vi "Get 3D Live Position Offset.vi"(3 "Mode":T5, 5 "Traverse line In":T2 {"Carrier_2 Q (l/min)" format="%#.2f"; "Row Duration (mins)" format="%#.1f"; "Row No" min=0; "Trace Gas Concentration (%)" min=0.0 format="%#_4f"; "Carrier_1 Q (l/min)" format="%#.2f"; "Tunnel Speed" format="%#.2f"; "Start X" format="%#.2f"; "Start Y" format="%#.2f"; "Start Z" format="%#.2f"; "End X" format="%#.2f"; "End Y" format="%#.2f"; "End Z" format="%#.2f"; "Averaging time (min)" min=0.0 format="%#.2f"}) -> (0 "Error Message":string, 1 "Status":T1, 2 "Traverse line Out":T2 {"Carrier_2 Q (l/min)" format="%#.2f"; "Row Duration (mins)" format="%#.1f"; "Row No" min=0; "Trace Gas Concentration (%)" min=0.0 format="%#_4f"; "Carrier_1 Q (l/min)" format="%#.2f"; "Tunnel Speed" format="%#.2f"; "Start X" format="%#.2f"; "Start Y" format="%#.2f"; "Start Z" format="%#.2f"; "End X" format="%#.2f"; "End Y" format="%#.2f"; "End Z" format="%#.2f"; "Averaging time (min)" min=0.0 format="%#.2f"})   [LabVIEW 2017]
uses:
  Gen Trav/Traverse_cluster.ctl
  Gen Trav/Spacing.ctl
  Controls/Multi_run_mode.ctl
  Controls/User_Specific_mode.ctl
  Gen Trav/Multi_Run_Status.ctl
  Controls/Setup.ctl
  Controls/Save_Data.ctl
  Camera Server/Camera enum/Camera resolution.ctl
  Globals/Trav_pos_global.vi
  Globals/Meas_global.vi
panel:
  out "Vertical Offset":sgl
  # "X           Y            Z"
  # "Start"
  # "End"
  # "X           Y            Z"
  # "Start"
  # "End"
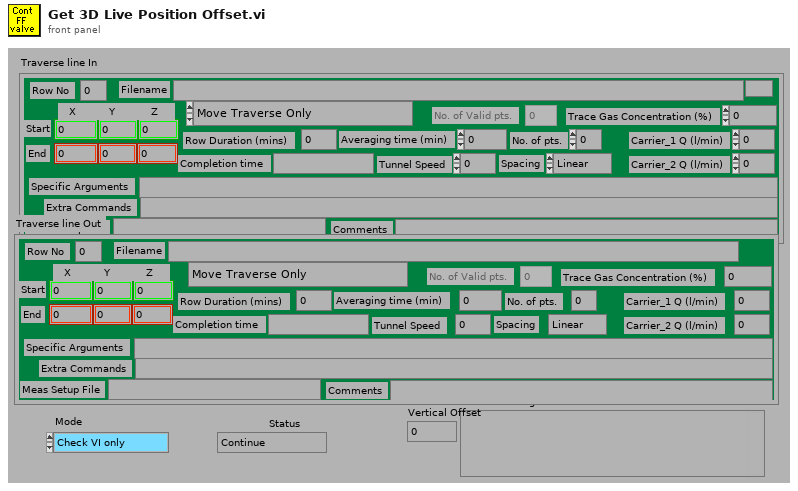
[diagram p1: front panel]
types:
  T1 = typedef "Multi_Run_Status.ctl" = enum16{"Continue", "Continue with Error", "Jump to Next Point", "Jump to Next Row", "Jump To Fall Back", "Terminate Run"}
  T2 = typedef "Traverse_cluster.ctl" = cluster{"Start X":sgl, "Start Y":sgl, "Start Z":sgl, "End X":sgl, "End Y":sgl, "End Z":sgl, "No. of pts.":i32, "Spacing":T3, "Filename":path, "Tunnel Speed":dbl, "Averaging time (min)":dbl, "Extra Commands":string, "Carrier_1 Q (l/min)":dbl, "Carrier_2 Q (l/min)":dbl, "Trace Gas Concentration (%)":dbl, "Specific Arguments":string, "Comments":string, "Row No":i32, "Row Type Selector":T4, "Completion time":string, "Row Duration (mins)":dbl, "No. of Valid pts.":i32, "Meas Setup File":string}
  T3 = typedef "Spacing.ctl" = enum16{"Linear", "Log", "Gauss", "Specified", "N/A"}
  T4 = typedef "Multi_run_mode.ctl" = enum16{"Move Traverse Only", "Set Tunnel Speed Only", "Set Source Only", "Set Measurement Conditions", "Single Measurement", "Vertical Profile", "Lateral Profile", "Longitudinal Profile", "Explore Volume", "Multi-Axis Profile", "Auto Calibrate", "Meas Fast FID Bkgnd", "Check Beam Power", "Scanning Valve Measurement", "Run VI Named:", "Set ADAM Ch", "Wait (minutes)", "Send Message", "Synchronize With:", "Fall Back to this Row", "Turn Off Row Repeating", "Blank Row", "Traverse 3D Volume"}
  T5 = typedef "User_Specific_mode.ctl" = enum16{"Check VI only", "Run VI"}
  T6 = enum16{"To Traverse Coordinates", "To User Coordinates"}
  T7 = typedef "Save_Data.ctl" = enum16{"Save No Data", "Save Data"}
  T8 = typedef "Setup.ctl" = enum16{"Run Program", "Show Setup", "Save Current Setup", "Setup Front Panel"}
  T9 = typedef "Tunnel_Coordinates.ctl" = enum16{"Work in Tunnel Coordinates", "Work in Model Coordinates"}
  T10 = typedef "Status_Cluster.ctl" = cluster{"Status":T1, "Error Type":string, "Error Description":string}
  T11 = typedef "Camera resolution.ctl" = u8
  T12 = typedef "Analysis_info_cluster.ctl" = cluster{"Colour":u32, "Inst type":T13, "Inst name":string, "Symbol":string, "Code name":string, "Extra Info":string, "Inst Array":T14, "Extra Titles":string[], "Extra Values":string[], "U":dbl, "u^2":dbl, "u^3":dbl, "u^4":dbl, "Skew_u":dbl, "Kurt_u":dbl, "Sd Error in Mean":dbl, "% u'/U":dbl, "X":dbl, "Y":dbl, "Z":dbl, "Timescale integral Estimate":dbl, "Sd Error in Variance":dbl, "Calib File":path, "Calib Constants":dbl[], "Output Position":bool, "Full Stats":bool, "Av Sampling Rate":dbl, "Av No of Samples":dbl, "Total Meas Time (s)":dbl, "ADAM Ch Name":string, "Max value":dbl, "Min value":dbl}
  T13 = typedef "Inst_type.ctl" = enum16{"Propeller anemometer", "Raw voltage", "Pressure Transducer", "Pitot-static tube", "Preston tube", "Hot wire", "Cross wire 1", "Cross wire 2", "Generic Linear", "Generic Polynomial", "Generic BackPoly", "Fast FID", "Thermocouple", "Cold wire", "Pulsed Wire", "LDA Vel", "LDA Tran time", "LDA Arr time", "Microphone"}
  T14 = typedef "Instrument_Array.ctl" = enum16{"PWA", "LDA", "Analogue"}
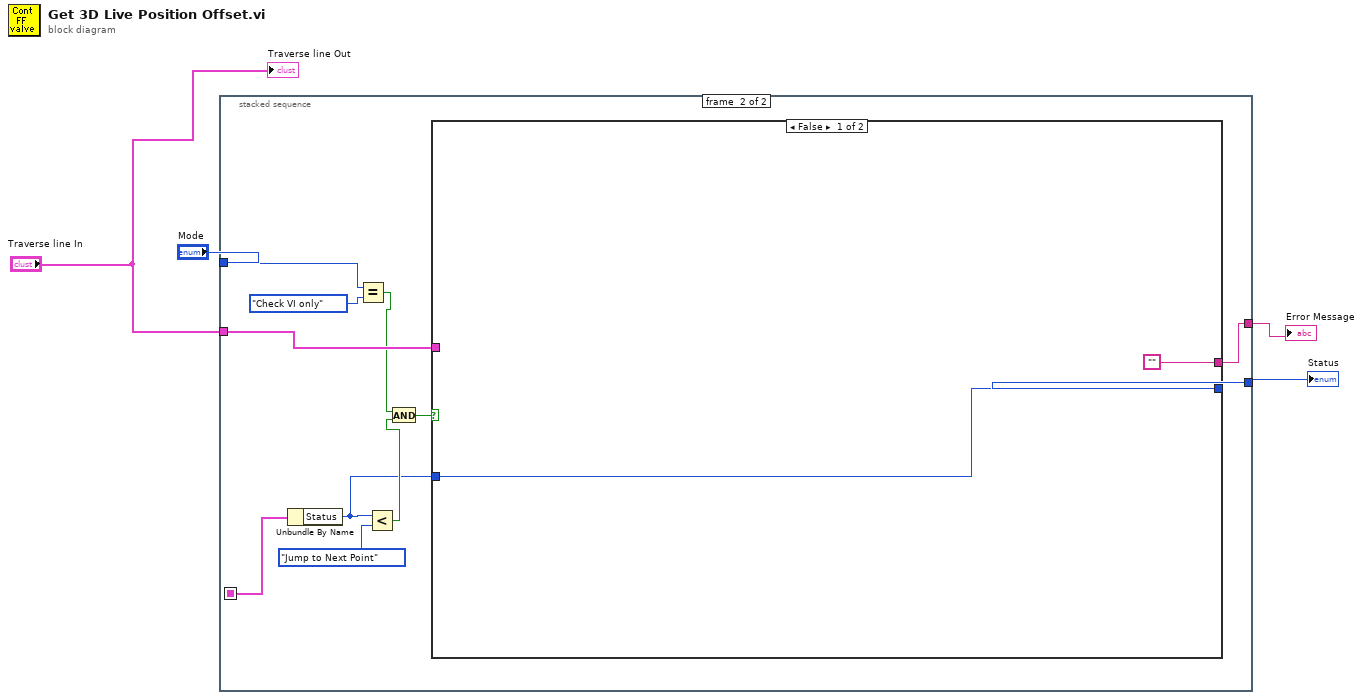
[diagram p0: block diagram]
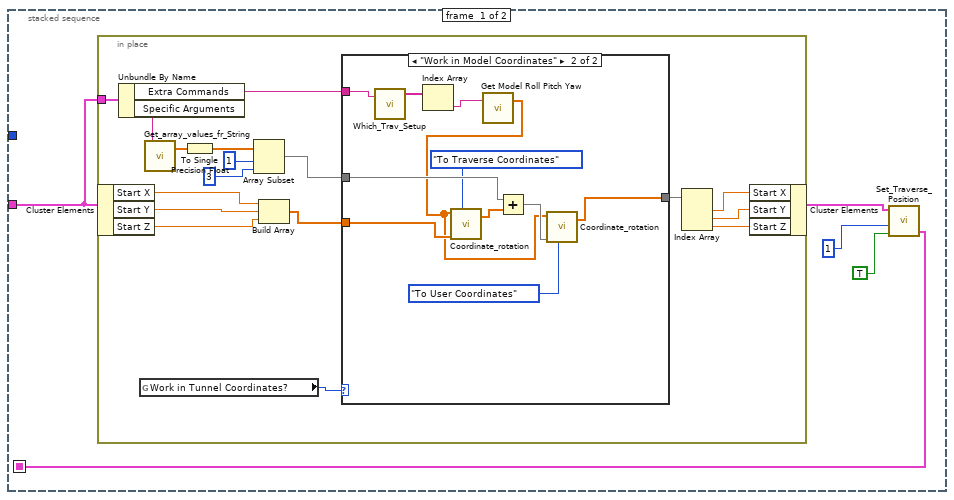
[diagram p2: hidden frame]
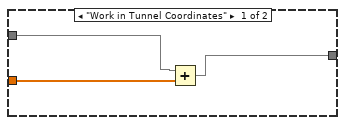
[diagram p3: hidden frame]
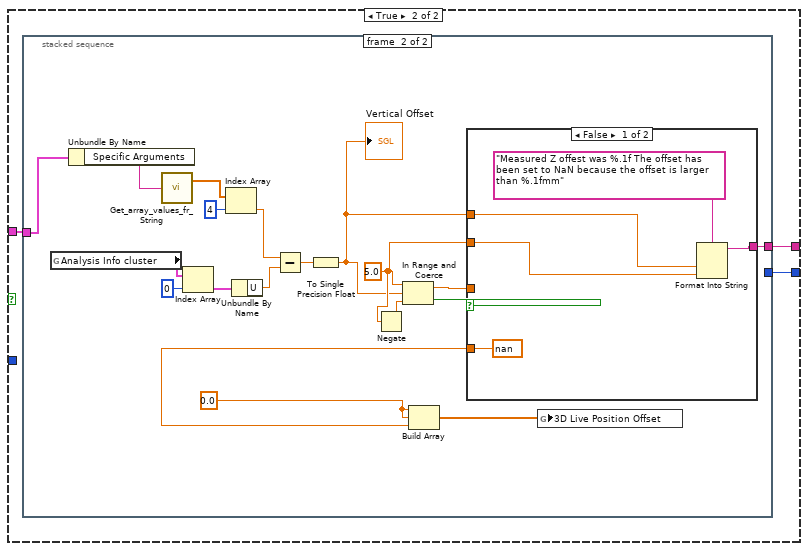
[diagram p4: hidden frame]
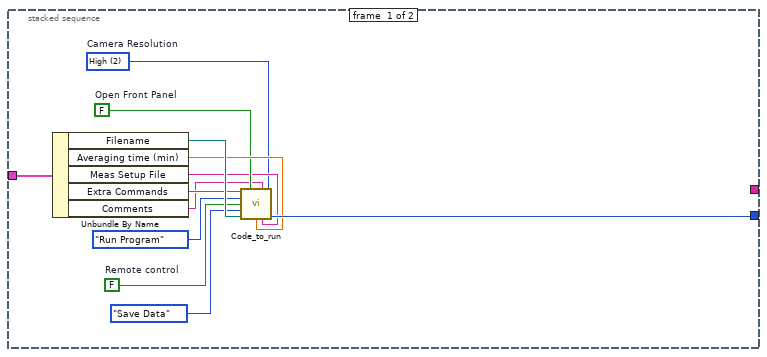
[diagram p5: hidden frame]
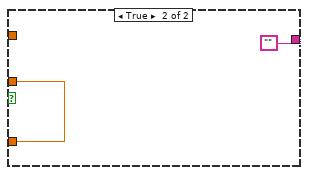
[diagram p6: hidden frame]
diagram:
  n1 = stacked-sequence {
    seq-local: [w6 _] -> [_ w50]
    tunnel: [_ w41] -> w4
    tunnel: "Traverse line In" -> [w5 w51]
    tunnel: "Mode" -> [_ w47]
    tunnel: [_ w43] -> w1
    frame #0 {
      n2 = in-place {
        in-place-border: w5 -> [w12]
        n3 = in-place-cluster #1(w5) -> ("Start X"=w24:sgl, "Start Y"=w23:sgl, "Start Z"=w22:sgl)
        n4 = Unbundle By Name(w12) -> ("Extra Commands"=w10:string, "Specific Arguments"=w11:string)
        n5 = global read "Trav_pos_global.vi" "Work in Tunnel Coordinates?"() -> (w26:T9)
        n6 = call "Get_array_values_fr_String.vi"("String Value"=w11) -> ("Numeric Array"=w25:dbl[])  [unwired: 1 out]
        n7 = To Single Precision Float(number=w25) -> (single precision float=w14:sgl[])
        n8 = Array Subset(array=w14, index=1, length=3) -> (w20:sgl[])
        n9 = Build Array(w24, w23, w22) -> (w19:sgl[])
        n10 = case shown="\"Work in Model Coordinates\"" w26 {
          tunnel: w20 -> [w29 w38]
          tunnel: w19 -> [w28 w40]
          tunnel: [w27 w36] -> w18
          tunnel: w10 -> [_ w31]
          frame "Work in Tunnel Coordinates" {
            n11 = Add(x=w29, y=w28) -> (x+y=w27:sgl[])
          }
          frame "Work in Model Coordinates" {
            n12 = call "Which_Trav_Setup.vi"("Extra Command String"=w31) -> ("Traverse Setups"=w33:string[])  [unwired: 1 in, 2 out]
            n13 = Index Array(array=w33) -> (element=w32:string)  [unwired: 1 in]
            n14 = call "Get Model Roll Pitch Yaw.vi"("Traverse Name"=w32) -> ("Model:    Roll        Pitch         Yaw  (deg)"=w30:sgl[])  [unwired: 1 in, 1 out]
            n15 = call "Coordinate_rotation.vi"("Roll-Pitch-Yaw"=w30, "Input Position"=w40, "Mode"=T6."To Traverse Coordinates") -> ("Output Position"=w39:sgl[])  [unwired: 2 in, 1 out]
            n16 = Add(x=w38, y=w39) -> (x+y=w37:sgl[])
            n17 = call "Coordinate_rotation.vi"("Roll-Pitch-Yaw"=w30, "Input Position"=w37, "Mode"=T6."To User Coordinates") -> ("Output Position"=w36:sgl[])  [unwired: 2 in, 1 out]
          }
        }
        n18 = Index Array(array=w18) -> (element #1=w17:sgl, element #2=w16:sgl, element #3=w15:sgl)  [unwired: 3 in]
        n19 = in-place-cluster #1("Start X"=w17, "Start Y"=w16, "Start Z"=w15) -> (w7:T2)
      }
      n20 = call "Set_Traverse_Position.vi"("Last Part of Move?"=TRUE, "Currently on Point"=1, "Traverse line"=w7) -> ("Status Cluster"=w6:T10)  [unwired: 3 in]
    }
    frame #1 {
      n21 = Unbundle By Name(w50) -> ("Status"=w42:T1)
      n22 = Equal?(x=w47, y=User_Specific_mode."Check VI only" ("Mode")) -> (x = y?=w45:bool)
      n23 = Less?(x=w42, y=Multi_Run_Status."Jump to Next Point") -> (x < y?=w46:bool)
      n24 = And(x=w45, y=w46) -> (x .and. y?=w44:bool)
      n25 = case shown="False" w44 {
        tunnel: [w53 w56] -> w43
        tunnel: w51 -> [_ w55]
        tunnel: w42 -> [w53 _]
        tunnel: ["" w54] -> w41
        frame False {
        }
        frame True {
          n26 = stacked-sequence {
            tunnel: [w68 _] -> w56
            tunnel: w55 -> [w57 w71]
            tunnel: [_ w69] -> w54
            frame #0 {
              w58 = T11 2 items=["Low", "Med.", "High", "Max."]  # Camera Resolution
              w64 = FALSE  # Open Front Panel
              w66 = FALSE  # Remote control
              n27 = Unbundle By Name(w57) -> ("Filename"=w67:path, "Averaging time (min)"=w65:dbl, "Meas Setup File"=w61:string, "Extra Commands"=w60:string, "Comments"=w59:string)
              n28 = call "Code_to_run.vi"("Extra command String"=w60, "Open Front Panel"=w64, "Current Row Comments"=w59, "Camera Resolution"=w58, "setup"=Setup."Run Program", "Remote control"=w66, "File"=Save_Data."Save Data", "Results Filename"=w67, "Averaging time (min)"=w65, "Setup filename"=w61) -> ("Status"=w68:T1)  [unwired: 2 in, 3 out]
            }
            frame #1 {
              w72 = sgl 5.0 ("upper limit")
              w78 = sgl 0.0
              n29 = global read "Meas_global.vi" "Analysis Info cluster"() -> (w87:T12[])
              n30 = Unbundle By Name(w71) -> ("Specific Arguments"=w84:string)
              n31 = call "Get_array_values_fr_String.vi"("String Value"=w84) -> ("Numeric Array"=w82:dbl[])  [unwired: 1 out]
              n32 = Index Array(array=w87, index=0) -> (element=w85:T12)
              n33 = Index Array(array=w82, index=4) -> (element=w81:dbl)
              n34 = Unbundle By Name(w85) -> ("U"=w80:dbl)
              n35 = Subtract(x=w81, y=w80) -> (x-y=w77:dbl)
              n36 = To Single Precision Float(number=w77) -> (single precision float=w70:sgl)
              "Vertical Offset" <- w70
              n37 = Negate(x=w72) -> (-x=w76:sgl)
              n38 = In Range and Coerce(upper limit=w72, x=w70, lower limit=w76) -> (coerced(x)=w74:sgl, In Range?=w75:bool)
              n39 = case shown="False" w75 {
                tunnel: w70 -> [w92 _]
                tunnel: w74 -> [_ w93]
                tunnel: [w90 ""] -> w69
                tunnel: [sgl nan ("upper limit") w93] -> w73
                tunnel: w72 -> [w88 _]
                frame False {
                  n40 = Format Into String(format string="Measured Z offest was %.1f The offset has  been set to NaN because the offset is larger than %.1fmm", w92, w88) -> (resulting string=w90:string)  [unwired: 2 in, 1 out]
                }
                frame True {
                }
              }
              n41 = Build Array(w78, w78, w73) -> (w79:sgl[])
              n42 = global write "Trav_pos_global.vi" "3D Live Position Offset"(w79) -> ()
            }
          }
        }
      }
    }
  }
  "Error Message" <- w4
  "Status" <- w1
  "Traverse line Out" <- "Traverse line In"
